vi "Design a Floating-Point Filter Part 3.vi"() -> ()   [LabVIEW 2023]
doc: "Part 3 of the Designing a Floating-Point Filter tutorial."
uses:
  <vilib>/addons/Digital Filter Design/Process.llb/DFD Filtering (Array).vi
  <vilib>/addons/Digital Filter Design/NI_DigFilterLicensed.lvlib
panel:
  out "Waveform Graph":dbl[][](graph)
  out "Magnitude Response":dynamicdata(graph) caption="magnitude"
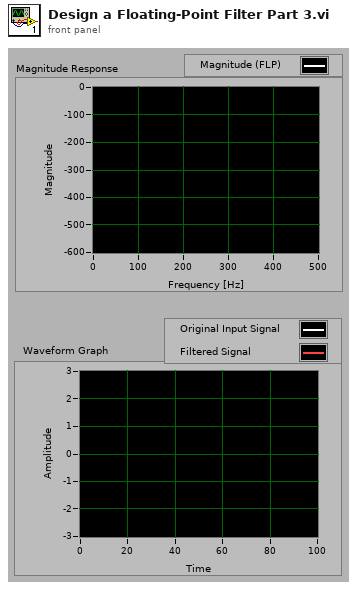
[diagram p1: front panel]
types:
  T1 = typedef "NI_DigFilterLicensed.lvlib/DFD Filter Obj.ctl" = cluster{"mSRate_Fs":dbl, "mSRate_Version":string, "mSRate_Comments":string, "mSRate_OrgCoef":T2, "mSRate_CurCoef":T2, "mSRate_Quantized?":bool, "mSRate_QCoef":T2, "mSRate_QSettings":T4[], "mSRate_Order":i32, "mSRate_Scaling":cluster{"mSRate_ScaleByPowerOf2?":bool, "mSRate_ScaleType":T6}}
  T2 = typedef "NI_DigFilterLicensed.lvlib/DFD Filter Coef.ctl" = cluster{"type":T3, "gain":dbl, "coef a (k)":dbl[], "coef b (v)":dbl[]}
  T3 = typedef "NI_DigFilterLicensed.lvlib/DFD Filter Structure Type Selector.ctl" = enum16{"Undefined", "FIR Direct Form", "FIR Direct Form Transposed", "FIR Symmetric", "FIR Antisymmetric", "IIR Direct Form I", "IIR Direct Form I Transposed", "IIR Direct Form II", "IIR Direct Form II Transposed", "IIR Cascaded Second Order Sections Form I", "IIR Cascaded Second Order Sections Form I Transposed", "IIR Cascaded Second Order Sections Form II", "IIR Cascaded Second Order Sections Form II Transposed", "Lattice Allpass (basic sections)", "Lattice Allpass (one multiplier sections)", "Lattice Allpass (normalized sections)", "Lattice AR (basic sections)", "Lattice AR (one multiplier sections)", "Lattice AR (normalized sections)", "Lattice MA (minimum phase)", "Lattice MA (maximum phase)", "Lattice ARMA (basic sections)", "Lattice ARMA (one multiplier sections)", "Lattice ARMA (normalized sections)"}
  T4 = typedef "NI_DigFilterLicensed.lvlib/dfd_Internal Quantization Settings.ctl" = cluster{"source":T5, "wl":i16, "iwl":i16, "overflow mode":enum16{"Saturation", "Wrap"}, "rounding mode":enum16{"Nearest", "Truncation"}, "signed?":bool}
  T5 = typedef "NI_DigFilterLicensed.lvlib/dfd_Internal Quantization Srcs.ctl" = u16
  T6 = typedef "NI_DigFilterLicensed.lvlib/DFD Coef Norm Type.ctl" = enum16{"No Norm", "Time Domain 1-Norm", "Time Domain 2-Norm", "Time Domain Inf-Norm"}
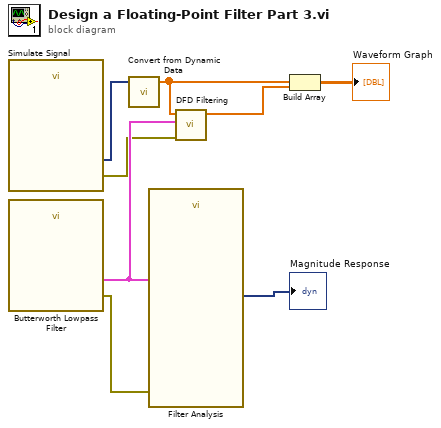
[diagram p0: block diagram]
diagram:
  n1 = call "Simulate Signal"() -> ("Sine with Gaussian Noise"=w6:dynamicdata, "error out"=w2:errorcluster)  [unwired: 8 in, 6 out]
  n2 = call "Butterworth Lowpass Filter"() -> ("error out"=w1:errorcluster, "filter out"=w7:T1)  [unwired: 1 in, 9 out]
  n3 = call "Convert from Dynamic Data"("Dynamic Data Type"=w6) -> ("Array"=w5:dbl[])  [unwired: 3 out]
  n4 = call "Filter Analysis"("error in (no error)"=w1, "filter in"=w7) -> ("magnitude"=→"Magnitude Response":dynamicdata)  [unwired: 9 out]
  n5 = call-poly <vilib>:"DFD Filtering.vi"("error in (no error)"=w2, "filter"=w7, "signal in"=w5) -> ("signal out"=w4:dbl[])  [unwired: 1 in, 7 out]
  n6 = Build Array "Build Array"(w5, w4) -> (→"Waveform Graph":dbl[][])
